vi "Read Serial Port.vi"(2 "error in (no error)":errorcluster, 3 "baud rate":u32=115200, 4 "Bluetooth Port":refnum<visa-resource-name>) -> (0 "error out":errorcluster, 1 "Output Data":string[](array[string]))   [LabVIEW 2015]
uses:
  <vilib>/Instr/_visa.llb/VISA Configure Serial Port (Instr).vi
panel:
  in  "Save to file":bool
  out "read buffer":string
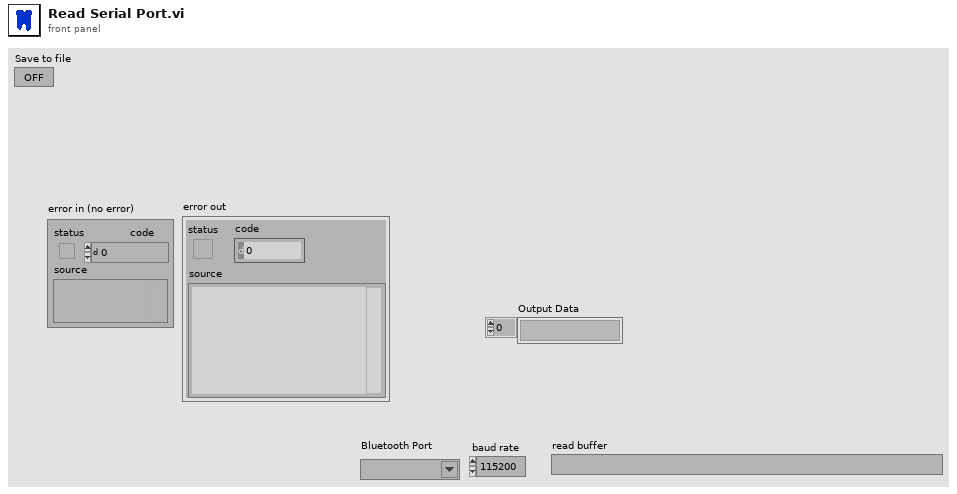
[diagram p1: front panel]
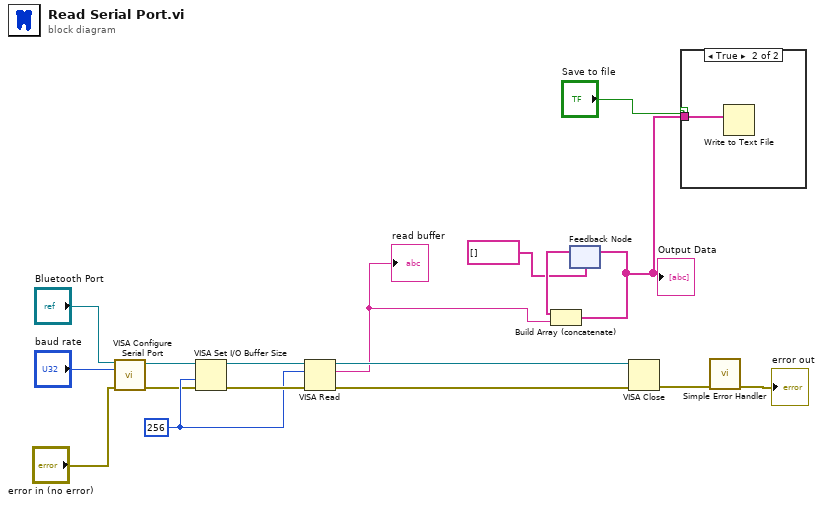
[diagram p0: block diagram]
diagram:
  w12 = u32 256 ("size (4096)")
  n1 = call-poly "VISA Configure Serial Port"("VISA resource name"="Bluetooth Port", "baud rate (9600)"="baud rate", "error in (no error)"="error in (no error)") -> ("VISA resource name out"=w15:refnum<visa-resource-name>, "error out"=w6:errorcluster)  [unwired: 11 in]
  n2 = VISA Set I/O Buffer Size(VISA resource name=w15, size (4096)=w12, error in (no error)=w6) -> (VISA resource name out=w14:refnum<visa-resource-name>, error out=w13:errorcluster)  [unwired: 1 in]
  n3 = VISA Read(VISA resource name=w14, byte count=w12, error in (no error)=w13) -> (VISA resource name out=w11:refnum<visa-resource-name>, read buffer=w2:string, error out=w10:errorcluster)  [unwired: 1 out]
  "read buffer" <- w2
  n4 = feedback #1(string[] []) -> (w3:string[])
  n5 = Build Array (concatenate)(w3, w2) -> (w5:string[])
  "Output Data" <- w5
  n6 = feedback-in #1(w5) -> ()
  n7 = VISA Close(VISA resource name=w11, error in (no error)=w10) -> (error out=w9:errorcluster)
  n8 = case shown="True" "Save to file" {
    tunnel: w5 -> [_ w18]
    frame False {
    }
    frame True {
      n9 = Write to Text File(text=w18) -> ()  [unwired: 3 in, 3 out]
    }
  }
  n10 = call <vilib>:"Simple Error Handler.vi"("error in (no error)"=w9) -> ("error out"=→"error out":errorcluster)  [unwired: 4 in, 4 out]
